vi "FlushBuffer.vi"(8 "error in (no error)":errorcluster, 10 "Mask":T1=16 items=["Flush Receive Buffer"=16, "Write Transmit Buffer to Device"=32, "Flush Receive Buffer (No I/O)"=64, "Flush Transmit Buffer"=128], 11 "Serial Controller in":refnum<class "Serial Controller.lvclass">) -> (0 "error out":errorcluster, 3 "Serial Controller out":refnum<class "Serial Controller.lvclass">)   [LabVIEW 2011, in "Serial Controller.lvclass"]
uses:
  Serial Controller.lvclass
  <vilib>/Instr/_visa.llb/VISA Flush IO Buffer Mask.ctl
  Serial Controller.lvclass/Serial Controller.ctl
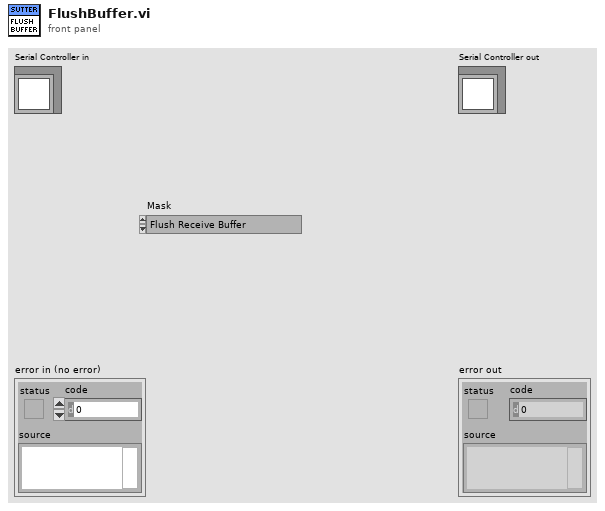
[diagram p1: front panel]
types:
  T1 = typedef "VISA Flush IO Buffer Mask.ctl" = u16
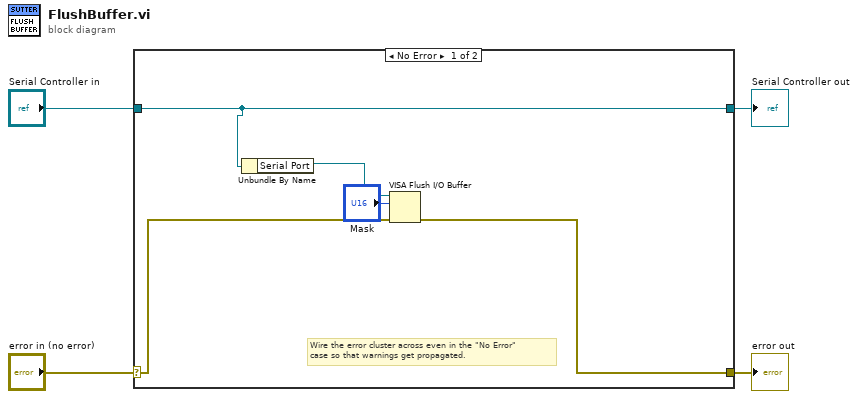
[diagram p0: block diagram]
diagram:
  n1 = case shown="No Error" "error in (no error)" {
    selector: "error in (no error)" -> [w7 w11]
    tunnel: [w6 w11] -> w3
    tunnel: [w9 w10] -> w1
    tunnel: "Serial Controller in" -> [w9 w10]
    frame No Error {
      # "Wire the error cluster across even in the \"No Error\"\ncase so that warnings get propagated."
      n2 = Unbundle By Name(w9) -> ("Serial Port"=w8:refnum<visa-resource-name>)
      n3 = VISA Flush I/O Buffer(VISA resource name=w8, mask (16)="Mask", error in (no error)=w7) -> (error out=w6:errorcluster)  [unwired: 1 out]
    }
    frame Error {
    }
  }
  "error out" <- w3
  "Serial Controller out" <- w1
